vi "WriteToUAv4.vi"() -> ()   [LabVIEW 2019]
uses:
  <vilib>/DAQmx/write.llb/DAQmx Write (Analog DBL 1Chan 1Samp).vi
  <vilib>/DAQmx/read.llb/DAQmx Read (Analog DBL 1Chan 1Samp).vi
  <vilib>/DAQmx/miscellaneous.llb/DAQmx Fill In Error Info.vi
  <vilib>/OPCUA/NI OPC UA Client.lvlib
panel:
  out "T_Airheater[C]":dbl
  in  "Tab Control":enum32{"Measurement", "OPC UA settings"}(tab)
  out "u_manual[V]":dbl format="%#_3g"
  out "Setpoint[C]":dbl=27.040816326530614 format="%#_4g"
  out "Temperature[C]":dbl=27.05378604137692 format="%#_4g"
  out "Thermometer[C]":dbl(slide)=27.054253878408307 scale=-10.0..50.0
  out "Thermometer[F]":dbl(slide)=80.69765698113495 scale=14.0..122.0
  out "Temperature[F]":dbl=80.69765698113495 format="%#_4g"
  in  "SetPoint [C]":dbl(slide)=23.979591836734695 scale=20.0..50.0
  in  "ON:Manual mode":bool caption="Manual/Automatic"
  in  "PI-parameters":cluster{"Kp":dbl, "Ti[s]":dbl}={"Kp"=1.46, "Ti[s]"=8.85}
  in  "u_manual[V]":dbl(slide) scale=0.0..5.0 scale format="%#_3g"
  in  "Node Id(temperature)":string="ns=2;s=Process Data.Temperature"
  in  "server endpoint URL":string="opc.tcp://Edv:49580"
  in  "security policy":T1
  in  "Node Id(setpoint)":string="ns=2;s=Setpoint"
  out "Temperature  Chart":T2(graph)
  out "Control Signal Chart":dbl(graph)=1.3296076034482445
  in  "stop":bool
  # "OFF:Automatic mode"
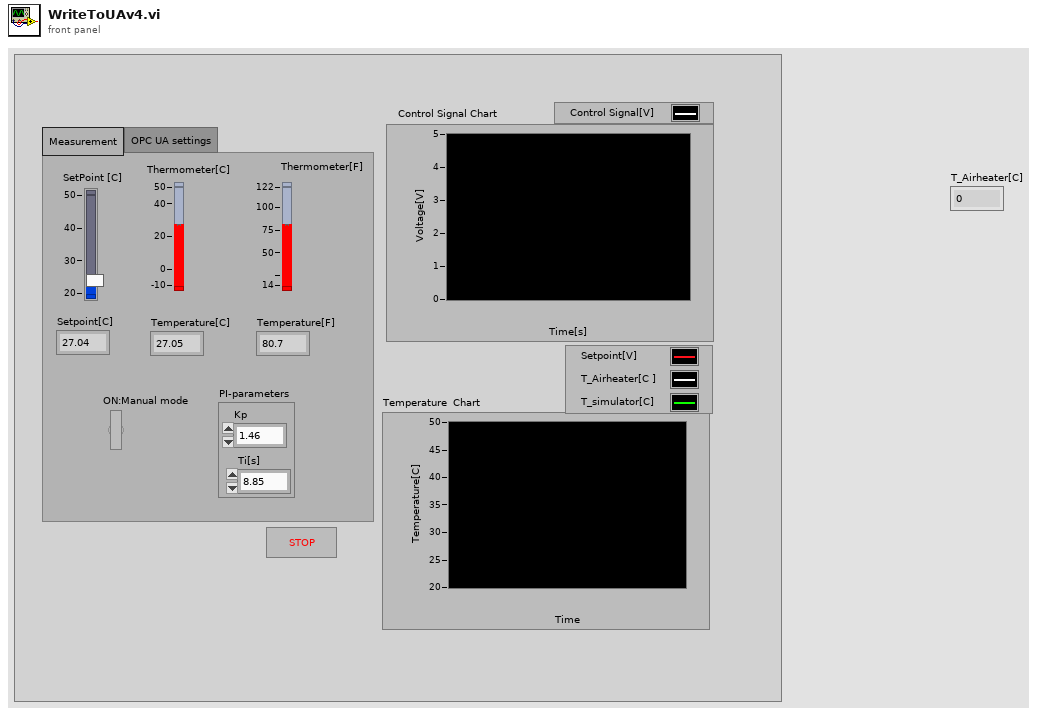
[diagram p1: front panel]
types:
  T1 = cluster{"message mode":enum16{"None", "Sign", "Sign and Encrypt"}, "security":enum16{"Basic256", "Basic128Rsa15"}}
  T2 = cluster{"SetPoint [C]":dbl, "T_Blackbox[C]":dbl, "Temperature[C]":dbl}
  T3 = cluster{"SetPoint [C]":dbl, "T_Blackbox[C]":dbl, "Temperature[C]":dbl}[]
  T4 = typedef "OPC UA Client Refnum.ctl" = refnum<k21>
  T5 = cluster{"SetPoint [C]":dbl, "T_Airheater[C]":dbl, "Temperature[C]":dbl}
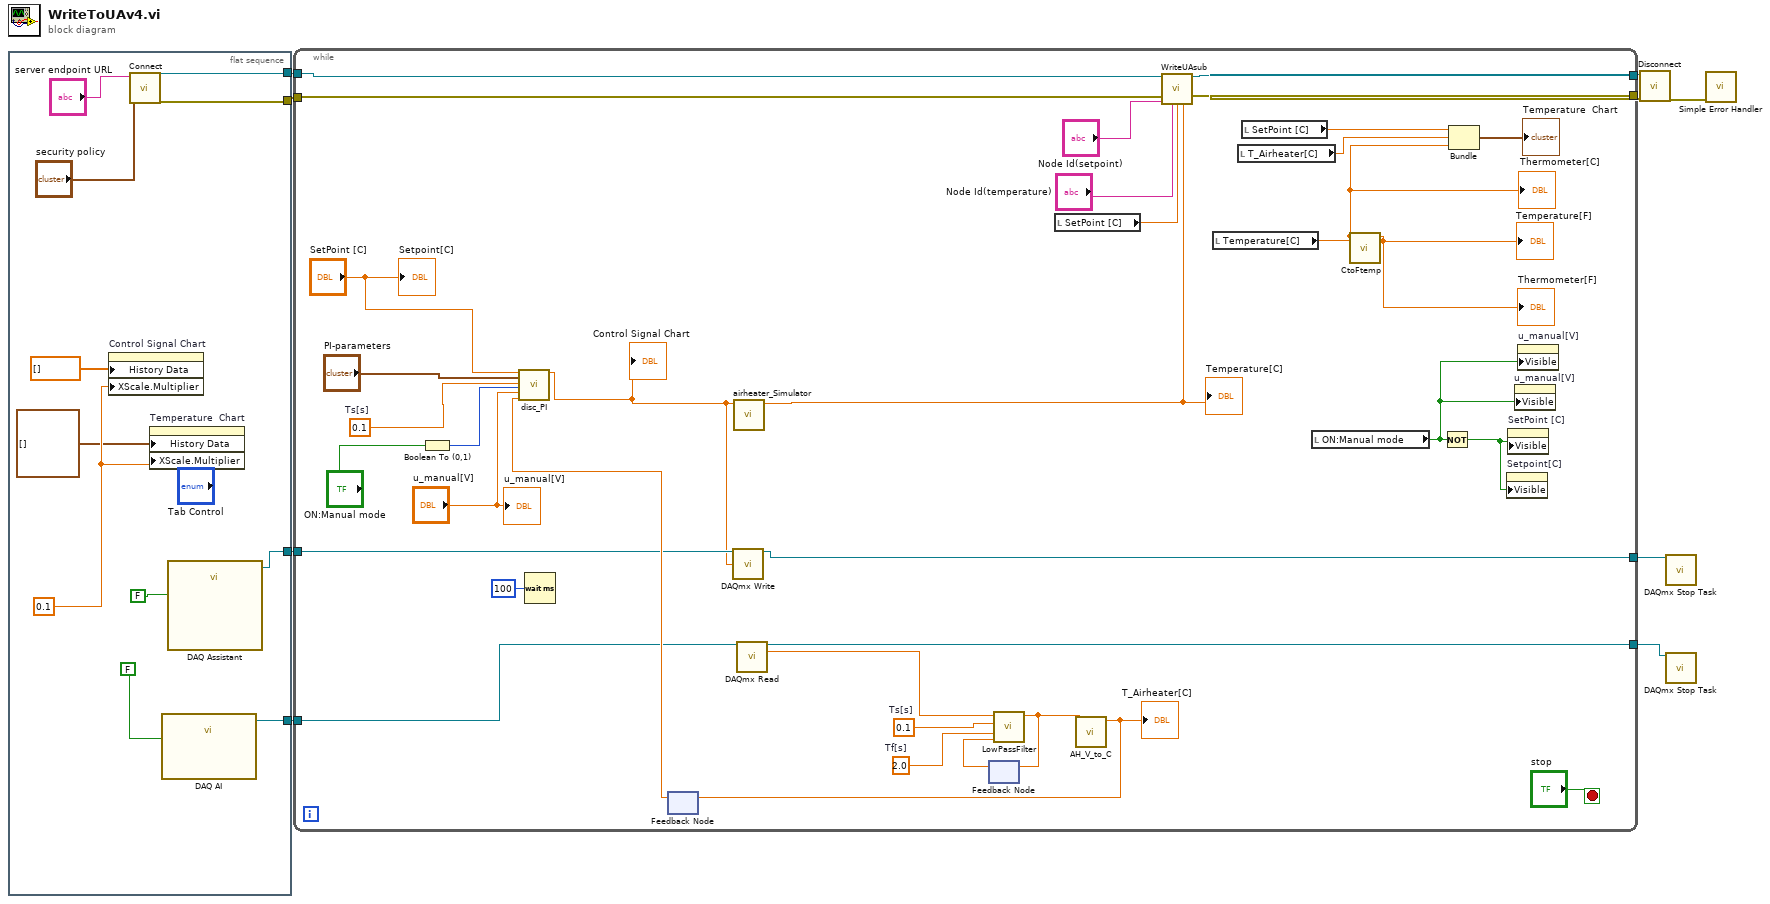
[diagram p0: block diagram]
diagram:
  n1 = flat-sequence {
    tunnel: [w18] -> w7
    tunnel: [w17] -> w6
    tunnel: [w11] -> w4
    tunnel: [w10] -> w3
    frame #0 {
      w15 = 0.1
      n2 = property on="Control Signal Chart" class="WFChart (strict)"("History Data"=dbl[] [], "XScale.Multiplier"=w15) -> ()  [unwired: 2 in, 2 out]
      n3 = call <vilib>:"Connect.vi"("security policy"="security policy", "server endpoint URL"="server endpoint URL") -> ("error out"=w18:errorcluster, "OPC UA client refnum out"=w17:T4)  [unwired: 7 in, 1 out]
      n4 = property on="Temperature  Chart" class="WFChart (strict)"("History Data"=T3 [], "XScale.Multiplier"=w15) -> ()  [unwired: 2 in, 2 out]
      n5 = call "DAQ AI"("stop (T)"=FALSE) -> ("task out"=w11:refnum<k21>)  [unwired: 16 in, 2 out]
      n6 = call "DAQ Assistant"("stop (T)"=FALSE) -> ("task out"=w10:refnum<k21>)  [unwired: 17 in, 1 out]
    }
  }
  n7 = while {
    tunnel: [w52] -> w8
    tunnel: w6 -> [w53]
    tunnel: w7 -> [w51]
    tunnel: [w48] -> w5
    tunnel: w4 -> [w25]
    tunnel: w3 -> [w24]
    tunnel: [w23] -> w2
    tunnel: [w22] -> w1
    stop <- "stop" stop-if-true
    w31 = 0.1  # Ts[s]
    w28 = 2.0  # Tf[s]
    w43 = 0.1  # Ts[s]
    n8 = Boolean To (0,1)(Boolean="ON:Manual mode") -> (0, 1=w45:i16)
    n9 = Wait (ms)(milliseconds to wait=u32 100) -> ()  [unwired: 1 out]
    n10 = feedback #1() -> (w46:dbl)  [unwired: 1 in]
    n11 = call "disc_PI.vi"("y_ref"="SetPoint [C]", "PISettiings"="PI-parameters", "Ts"=w43, "manual"=w45, "u_man"="u_manual[V]", "y"=w46) -> ("u_k"=w21:dbl)  [unwired: 13 in]
    "Control Signal Chart" <- w21
    n12 = call-poly <vilib>:"DAQmx Write.vi"("task/channels in"=w24, "data"=w21) -> ("task out"=w23:refnum<k21>)  [unwired: 11 in, 2 out]
    n13 = call "airheater_Simulator.vi"("Control Signal [V]"=w21) -> ("T_out[C]"=w38:dbl)  [unwired: 10 in]
    "Temperature[C]" <- w38
    n14 = call-poly <vilib>:"DAQmx Read.vi"("task/channels in"=w25) -> ("task out"=w22:refnum<k21>, "data"=w27:dbl)  [unwired: 12 in, 1 out]
    n15 = feedback #2() -> (w29:dbl)  [unwired: 1 in]
    n16 = call "LowPassFilter.vi"("input variable"=w29, "Tf[s]"=w28, "Ts[s]"=w31, "u_k"=w27) -> ("output variable"=w30:dbl)  [unwired: 7 in]
    n17 = feedback-in #2(w30) -> ()
    n18 = local read "SetPoint [C]"() -> (w39:dbl)
    n19 = call "AH_V_to_C.vi"("Vin[1-5V]"=w30) -> ("Tout[C]"=w26:dbl)  [unwired: 10 in]
    "T_Airheater[C]" <- w26
    n20 = feedback-in #1(w26) -> ()
    n21 = call "WriteUAsub.vi"("OPC UA client refnum in"=w53, "error in (no error)"=w51, "SetpointID"="Node Id(setpoint)", "TemperatureID"="Node Id(temperature)", "Setpoint[C]"=w39, "Temperature[C]"=w38) -> ("OPC UA client refnum out"=w52:T4, "error out"=w48:errorcluster)  [unwired: 8 in]
    n22 = local read "Temperature[C]"() -> (w35:dbl)
    "Thermometer[C]" <- w35
    n23 = local read "T_Airheater[C]"() -> (w34:dbl)
    n24 = local read "SetPoint [C]"() -> (w36:dbl)
    n25 = local read "ON:Manual mode"() -> (w40:bool)
    n26 = call "CtoFtemp.vi"("Numeric in"=w35) -> ("Numeric out"=→"Thermometer[F]" →"Temperature[F]":dbl)  [unwired: 10 in]
    n27 = Not(x=w40) -> (.not. x?=w42:bool)
    n28 = Bundle("SetPoint [C]"=w36, "T_Airheater[C]"=w34, "Temperature[C]"=w35) -> (→"Temperature  Chart":T5)  [unwired: 1 in]
    n29 = property on="Setpoint[C]" class="DigNum (strict)"("Visible"=w42) -> ()  [unwired: 2 in, 2 out]
    n30 = property on="SetPoint [C]" class="Slide (strict)"("Visible"=w42) -> ()  [unwired: 2 in, 2 out]
    n31 = property on="u_manual[V]" class="DigNum (strict)"("Visible"=w40) -> ()  [unwired: 2 in, 2 out]
    n32 = property on="u_manual[V]" class="Slide (strict)"("Visible"=w40) -> ()  [unwired: 2 in, 2 out]
    "Setpoint[C]" <- "SetPoint [C]"
    "u_manual[V]" <- "u_manual[V]"
  }
  n33 = call <vilib>:"Disconnect.vi"("error in (no error)"=w5, "OPC UA client refnum in"=w8) -> ("error out"=w9:errorcluster)  [unwired: 9 in]
  n34 = call <vilib>:"DAQmx Stop Task.vi"("task/channels in"=w2) -> ()  [unwired: 13 in, 2 out]
  n35 = call <vilib>:"DAQmx Stop Task.vi"("task/channels in"=w1) -> ()  [unwired: 13 in, 2 out]
  n36 = call <vilib>:"Simple Error Handler.vi"("error in (no error)"=w9) -> ()  [unwired: 4 in, 5 out]
